vi "save NM.vi"(6 "anno":string, 8 "Filtro":bool[](array[boolean]), 9 "MEMO NPSH":string[][][](array[string]), 10 "Array":refnum<vi>[](array[refnum]), 11 "Numero":string) -> (0 "error out":errorcluster)   [LabVIEW 2019]
uses:
  <vilib>/addons/database/Connection.llb/Conn Execute.vi
  <vilib>/addons/database/Recordset.llb/Rec Destroy - Connection.vi
  <vilib>/addons/database/NI_Database_API.lvlib
panel:
  out "seconds since 1Jan1904":timestamp
  out "transposed array":string[][](array[string])
  out "Completamento":string
  in  "error in (no error)":errorcluster
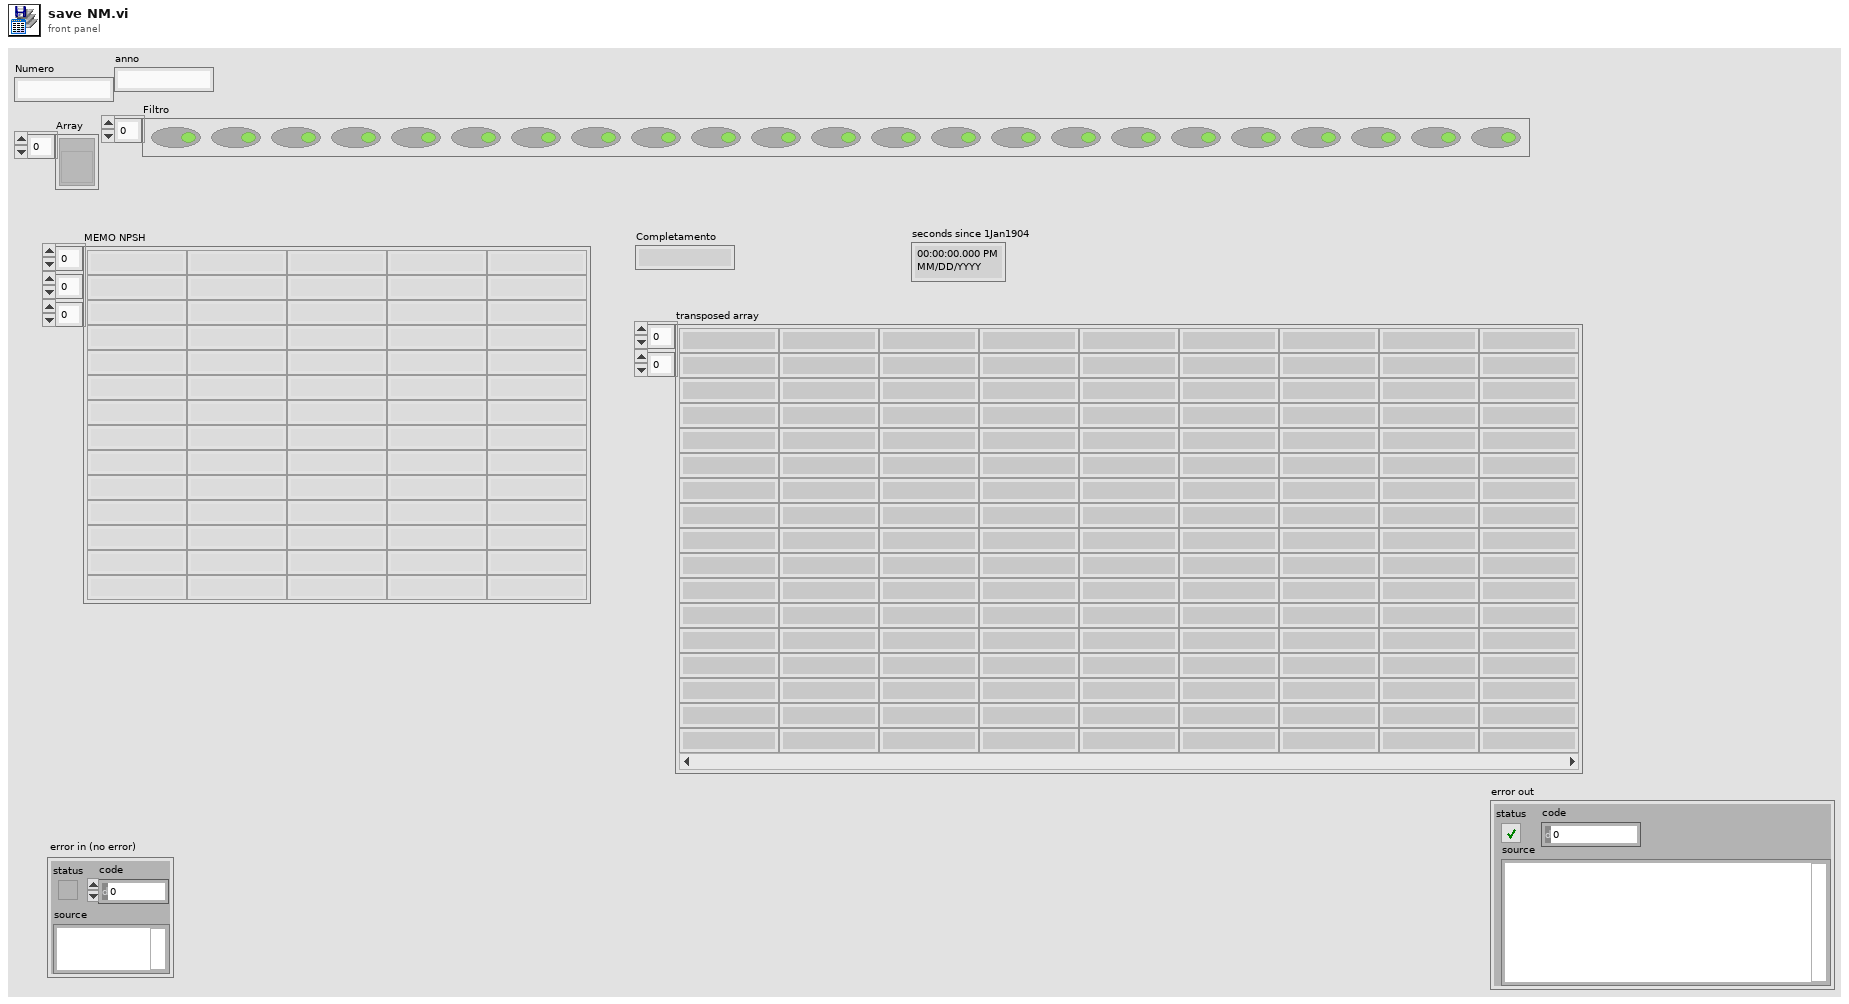
[diagram p1: front panel]
types:
  T1 = typedef "NI_Database_API.lvlib/Conn ObjectReference.ctl" = refnum<k1>
  T2 = typedef "NI_Database_API.lvlib/Rec ObjectReference.ctl" = refnum<k1>
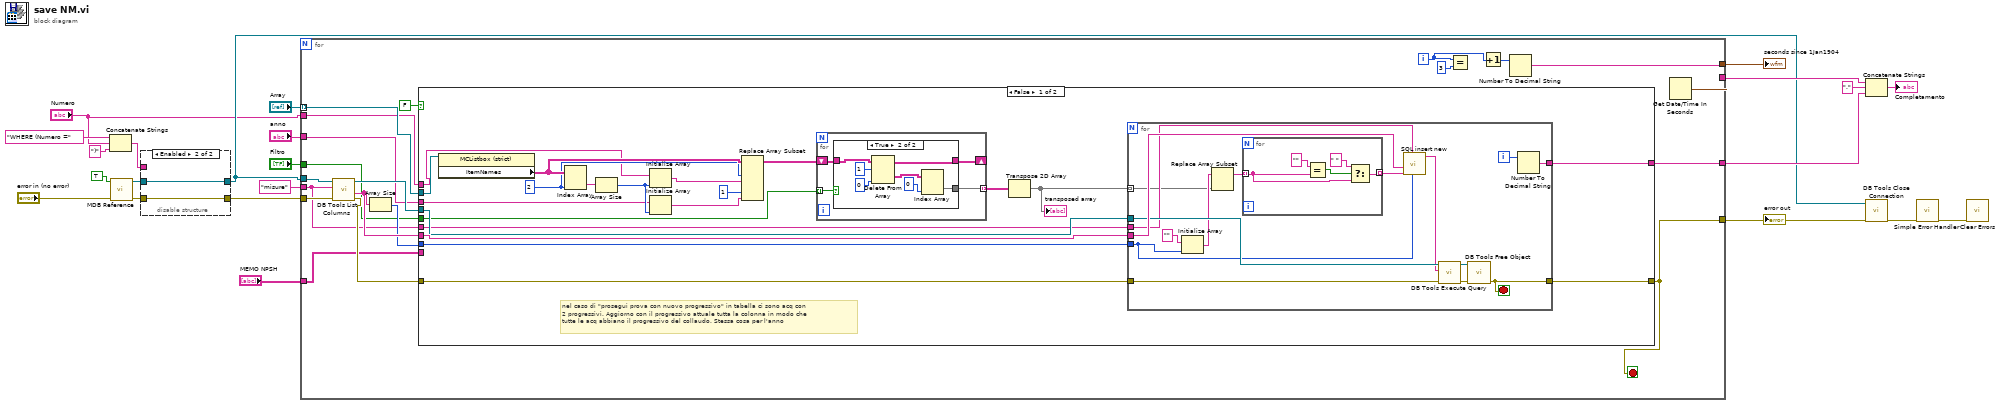
[diagram p0: block diagram]
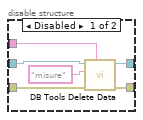
[diagram p2: hidden frame]
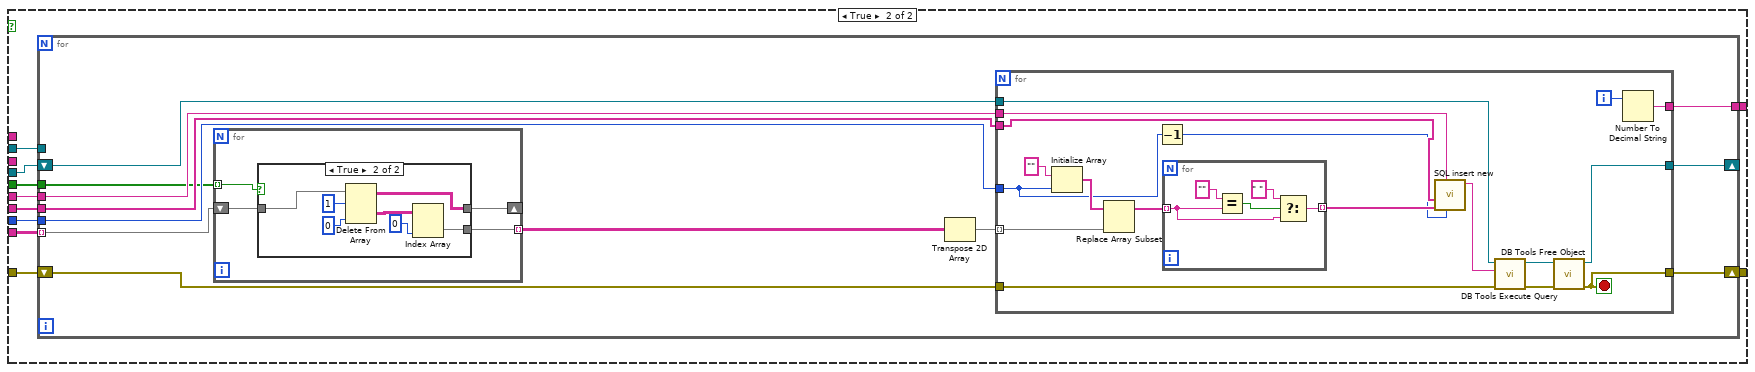
[diagram p4: hidden frame]
diagram:
  n1 = Concatenate Strings("WHERE (Numero =" ("condition"), "Numero", ")" ("string")) -> (w16:string)
  n2 = call "MDB Reference.vi"("error in (no error)"="error in (no error)", "Collaudi T/motori F"=TRUE ("NM?")) -> ("error out"=w17:errorcluster, "Refnum out"=w18:T1)  [unwired: 7 in, 1 out]
  n3 = disable-structure shown="Enabled" {
    disable-tunnel: w18 -> [w29 w31]
    disable-tunnel: w17 -> [w28 w30]
    disable-tunnel: w16 -> [w27 _]
    disable-tunnel: [w25 w31] -> w4
    disable-tunnel: [w24 w30] -> w15
    frame Disabled {
      n4 = call <vilib>:"DB Tools Delete Data.vi"("condition"=w27, "error in (no error)"=w28, "table"="misure", "connection reference"=w29) -> ("error out"=w24:errorcluster, "connection reference out"=w25:T1)  [unwired: 6 in]
    }
    frame Enabled {
    }
  }
  n5 = for {
    tunnel: "Array" -> [w51] mode=indexing
    tunnel: w4 -> [w50]
    tunnel: [w34] -> w3
    tunnel: w15 -> [w49]
    tunnel: "misure" ("table") -> [w44]
    tunnel: "MEMO NPSH" -> [w42]
    tunnel: "Filtro" -> [w41]
    tunnel: [w40] -> w10
    tunnel: [w37] -> w11
    tunnel: [w35] -> w8
    tunnel: "Numero" -> [w33]
    tunnel: "anno" -> [w32]
    i -> [w39]
    stop <- w34 stop-if-true
    n6 = call <vilib>:"DB Tools List Columns.vi"("error in (no error)"=w49, "table"=w44, "connection reference"=w50) -> ("error out"=w45:errorcluster, "columns"=w48:string[], "connection reference out"=w46:T1)  [unwired: 2 out]
    n7 = Array Size(array=w48) -> (size(s)=w47:i32)
    n8 = case shown="False" FALSE {
      tunnel: w51 -> [w72 w115]
      tunnel: [w71 w114] -> w34
      tunnel: w48 -> [w70 w113]
      tunnel: w47 -> [w69 w112]
      tunnel: w46 -> [w68 w111]
      tunnel: w45 -> [w67 w110]
      tunnel: w44 -> [w66 w109]
      tunnel: w42 -> [_ w108]
      tunnel: w41 -> [w64 w107]
      tunnel: [w65 w106] -> w40
      tunnel: w33 -> [w55 _]
      tunnel: w32 -> [w52 _]
      frame False {
        w60 = 2 ("disabled index (col)")
        # "nel caso di \"prosegui prova con nuovo progressivo\" in tabella ci sono acq con\n2 progressivi. Aggiorno con il progressivo attuale tutta la colonna in modo che\ntutte le acq abbiano il progressivo del collaudo. Stessa cosa per l'anno"
        n9 = property class="MCListbox (strict)"(reference=w72) -> ("ItemNames"=w61:string[][])  [unwired: 1 in, 2 out]
        n10 = Index Array(array=w61, index (col)=w60) -> (element=w58:string[])  [unwired: 1 in]
        n11 = Array Size(array=w58) -> (size(s)=w54:i32)
        n12 = Initialize Array(w55, w54) -> (w57:string[])
        n13 = Initialize Array(w52, w54) -> (w53:string[])
        n14 = Replace Array Subset(array=w61, new element #1=w57, index (col) #1=w60, new element #2=w53, index (col) #2=1 ("index (col)")) -> (w59:string[][])  [unwired: 2 in]
        n15 = for {
          shift-right: [w75] -> _
          shift-left: w59 -> [w76]
          tunnel: w64 -> [w74] mode=indexing
          tunnel: [w73] -> w63 mode=indexing
          n16 = case shown="True" w74 {
            tunnel: w76 -> [w77 w84]
            tunnel: [w77 w81] -> w75
            tunnel: [_ w79] -> w73
            frame False {
            }
            frame True {
              n17 = Delete From Array(array=w84, length=1, index (col)=0 ("disabled index (col)")) -> (deleted portion=w80:string[][], array with subset deleted=w81:string[][])  [unwired: 1 in]
              n18 = Index Array(array=w80, index (col)=0 ("index (row)")) -> (element=w79:string[])  [unwired: 1 in]
            }
          }
        }
        n19 = Transpose 2D Array(2D array=w63) -> (transposed array=w62:string[][])
        "transposed array" <- w62
        n20 = for {
          tunnel: w70 -> [w100]
          tunnel: w68 -> [w99]
          tunnel: w67 -> [w97]
          tunnel: [w89] -> w71
          tunnel: w69 -> [w85]
          tunnel: w66 -> [w90]
          tunnel: [w87] -> w65
          tunnel: w62 -> [w86] mode=indexing
          i -> [w88]
          stop <- w89 stop-if-true
          n21 = Initialize Array("", w85) -> (w93:string[])
          n22 = Replace Array Subset(array=w93, new element=w86) -> (w92:string[])  [unwired: 1 in]
          n23 = for {
            tunnel: w92 -> [w103] mode=indexing
            tunnel: [w101] -> w91 mode=indexing
            n24 = Equal?(x="", y=w103) -> (x = y?=w104:bool)
            n25 = Select(t=" ", s=w104, f=w103) -> (s? t:f=w101:string)
          }
          n26 = call "SQL insert new .vi"("Numeric 2"=w85, "Nome Tabella"=w90, "ArrayValoriCampi1D"=w91, "ArrayNomiCampi1D"=w100) -> ("output"=w98:string)  [unwired: 7 out]
          n27 = call-poly <vilib>:"DB Tools Execute Query.vi"("error in (no error)"=w97, "SQL query"=w98, "connection reference"=w99) -> ("error out"=w96:errorcluster, "recordset reference"=w95:T2)  [unwired: 5 in]
          n28 = call-poly <vilib>:"DB Tools Free Object.vi"("error in (no error)"=w96, "recordset reference"=w95) -> ("error out"=w89:errorcluster)  [unwired: 8 in, 1 out]
          n29 = Number To Decimal String(number=w88) -> (decimal integer string=w87:string)  [unwired: 1 in]
        }
      }
      frame True {
        n30 = for {
          tunnel: w115 -> [_]
          tunnel: w113 -> [w125]
          tunnel: w112 -> [w124]
          tunnel: w109 -> [w121]
          shift-right: [w127] -> _
          shift-left: w111 -> [w123]
          shift-right: [w126] -> w114
          shift-left: w110 -> [w122]
          tunnel: w108 -> [w118] mode=indexing
          tunnel: w107 -> [w119]
          tunnel: [w120] -> w106
          n31 = for {
            shift-right: [w130] -> _
            shift-left: w118 -> [w131]
            tunnel: w119 -> [w129] mode=indexing
            tunnel: [w128] -> w117 mode=indexing
            n32 = case shown="True" w129 {
              tunnel: w131 -> [w132 w139]
              tunnel: [w132 w136] -> w130
              tunnel: [_ w134] -> w128
              frame False {
              }
              frame True {
                n33 = Delete From Array(array=w139, length=1, index (col)=0 ("disabled index (col)")) -> (deleted portion=w135:string[][], array with subset deleted=w136:string[][])  [unwired: 1 in]
                n34 = Index Array(array=w135, index (col)=0 ("index (row)")) -> (element=w134:string[])  [unwired: 1 in]
              }
            }
          }
          n35 = Transpose 2D Array(2D array=w117) -> (transposed array=w116:string[][])
          n36 = for {
            tunnel: w125 -> [w157]
            tunnel: w123 -> [w156]
            tunnel: w122 -> [w154]
            tunnel: [w143] -> w126
            tunnel: [w151] -> w127
            tunnel: w124 -> [w146]
            tunnel: w121 -> [w144]
            tunnel: [w141] -> w120
            tunnel: w116 -> [w140] mode=indexing
            i -> [w142]
            stop <- w143 stop-if-true
            n37 = Initialize Array("", w146) -> (w149:string[])
            n38 = Replace Array Subset(array=w149, new element=w140) -> (w148:string[])  [unwired: 1 in]
            n39 = Decrement(x=w146) -> (x-1=w145:i32)
            n40 = for {
              tunnel: w148 -> [w160] mode=indexing
              tunnel: [w158] -> w147 mode=indexing
              n41 = Equal?(x="", y=w160) -> (x = y?=w161:bool)
              n42 = Select(t=" ", s=w161, f=w160) -> (s? t:f=w158:string)
            }
            n43 = call "SQL insert new .vi"("Numeric 2"=w145, "Nome Tabella"=w144, "ArrayValoriCampi1D"=w147, "ArrayNomiCampi1D"=w157) -> ("output"=w155:string)  [unwired: 7 out]
            n44 = call-poly <vilib>:"DB Tools Execute Query.vi"("error in (no error)"=w154, "SQL query"=w155, "connection reference"=w156) -> ("error out"=w153:errorcluster, "recordset reference"=w152:T2)  [unwired: 5 in]
            n45 = call-poly <vilib>:"DB Tools Free Object.vi"("error in (no error)"=w153, "recordset reference"=w152) -> ("error out"=w143:errorcluster, "connection reference"=w151:T1)  [unwired: 8 in]
            n46 = Number To Decimal String(number=w142) -> (decimal integer string=w141:string)  [unwired: 1 in]
          }
        }
      }
    }
    n47 = Equal?(x=w39, y=3) -> ()  [unwired: 1 out]
    n48 = Increment(x=w39) -> (x+1=w38:i32)
    n49 = Number To Decimal String(number=w38) -> (decimal integer string=w37:string)  [unwired: 1 in]
    n50 = Get Date/Time In Seconds() -> (seconds since 1Jan1904=w35:timestamp)
  }
  "error out" <- w3
  "seconds since 1Jan1904" <- w8
  n51 = Concatenate Strings(w11, "." ("string"), w10) -> (→"Completamento":string)
  n52 = call <vilib>:"DB Tools Close Connection.vi"("error in (no error)"=w3, "connection reference"=w4) -> ("error out"=w7:errorcluster)  [unwired: 5 in]
  n53 = call <vilib>:"Simple Error Handler.vi"("error in (no error)"=w7) -> ("error out"=w6:errorcluster)  [unwired: 4 in, 4 out]
  n54 = call <vilib>:"Clear Errors.vi"("error in (no error)"=w6) -> ()  [unwired: 5 in, 2 out]
